vi "Set Trigger Current Limit.vi"(8 "error in (no error)":errorcluster, 9 "Unit(A)":u16(ring) items=["A", "mA", "uA"], 10 "Current Limit":dbl format="%.2f", 11 "VISA resource name":refnum<visa-resource-name>) -> (0 "error out":errorcluster, 3 "VISA resource name out":refnum<visa-resource-name>)   [LabVIEW 2018, in "Keithley KE22xx Series.lvlib"]
doc: "Set the value of Triggered Current Limit."
uses:
  Keithley KE22xx Series.lvlib
panel:
  # "© 2012 Keithley Instruments, Inc. ALL RIGHTS RESERVED"
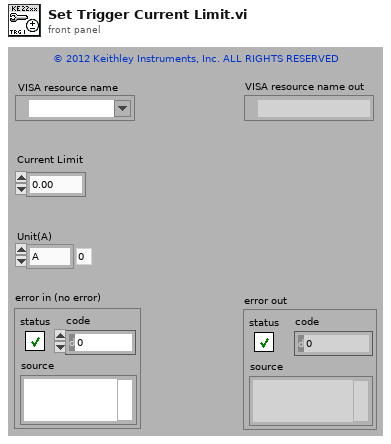
[diagram p1: front panel]
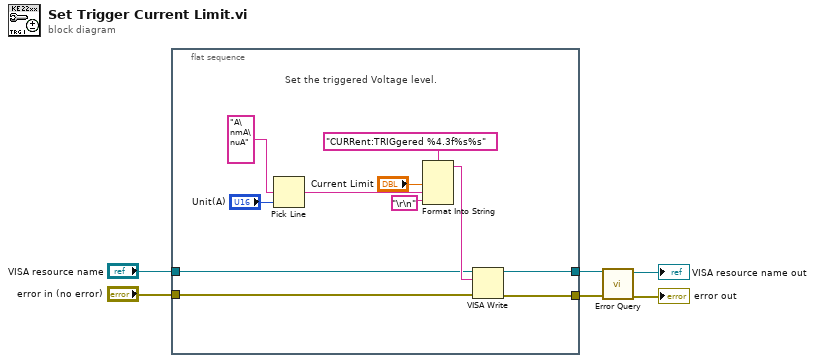
[diagram p0: block diagram]
diagram:
  n1 = flat-sequence {
    tunnel: "VISA resource name" -> [w10]
    tunnel: "error in (no error)" -> [w9]
    tunnel: [w8] -> w2
    tunnel: [w7] -> w1
    frame #0 {
      # "Set the triggered Voltage level."
      n2 = Pick Line(multi-line string="A\nmA\nuA", line index="Unit(A)") -> (output string=w13:string)  [unwired: 1 out]
      n3 = Format Into String(format string="CURRent:TRIGgered %4.3f%s%s", "Current Limit", w13, "\r\n") -> (resulting string=w17:string)  [unwired: 2 in, 1 out]
      n4 = VISA Write(VISA resource name=w10, write buffer=w17, error in (no error)=w9) -> (VISA resource name out=w8:refnum<visa-resource-name>, error out=w7:errorcluster)  [unwired: 1 out]
    }
  }
  n5 = call "Error Query.vi"("error in (no error)"=w1, "VISA resource name"=w2) -> ("error out"=→"error out":errorcluster, "VISA resource name out"=→"VISA resource name out":refnum<visa-resource-name>)  [unwired: 6 in, 2 out]
